vi "ConfigureDlg.vi"(8 "error in (no error)":errorcluster, 11 "RoomAlert in":refnum<class "RoomAlert.lvclass">) -> (0 "error out":errorcluster, 2 "Changed":bool, 3 "RoomAlert out":refnum<class "RoomAlert.lvclass">)   [LabVIEW 2018, in "SensorPlugins.lvlib" / "RoomAlert.lvclass"]
doc: "Configure the instrument using the provided panel and saves the instruments configuration to file, a new file, or cancels the entire operation."
uses:
  RoomAlert.lvclass
  C:/Program Files/National Instruments/LabVIEW 2018/user.lib/NIST/BaseClasses/BasePlugin_class/BasePlugin.lvclass
  TypeDefinitions/RoomAlertControls.ctl
  TypeDefinitions/MeasurementControls.ctl
  <userlib>/NIST/BaseClasses/BasePlugin_class/BasePlugin.lvclass/BasePlugin.ctl
  <userlib>/NIST/BaseClasses/BasePlugin_class/Accessors/Read PluginIniFilePath.vi
  <userlib>/NIST/BaseClasses/BasePlugin_class/Accessors/Write PluginIniFilePath.vi
  <vilib>/Utility/config.llb/NI_LVConfig.lvlib
panel:
  in  "Refresh Measurements Array":bool
  in  "MeasurementCluster":T1={"Measurement RefreshTime (ms)"=1000, "Measurement Name"="Sensor.RoomAlert0", "Timeout(ms)"=1000, "Amber Warning Light Configuration"={"Warning Temperture (Degrees C)"=0.0, "Temperature Delta (Degrees C/Minute)"=0.0, "Time Window (Minutes)"=0.0}} {"Amber Warning Light Configuration"."Time Window (Minutes)" min=0.0; "Timeout(ms)" min=5000; "Measurement RefreshTime (ms)" min=1000}
  in  "RoomAlert Device":T2 {"Measurements To Read Array" items=["Model ID", "Alarm Message", "Internal Temp F", "Internal Temp C", "Digital Sensor 1 Temp F", "Digital Sensor 1 Temp C", "Digital Sensor 2 Temp F", "Digital Sensor 2 Temp C", "Digital Sensor 3 Temp F", "Digital Sensor 3 Temp C", "Digital Switch 1", "Digital Switch 2", "Digital Switch 3", "Digital Switch 4", "Relay"]}
  in  "btnSaveAs":bool
  in  "btnSave":bool
  in  "btnCancel":bool
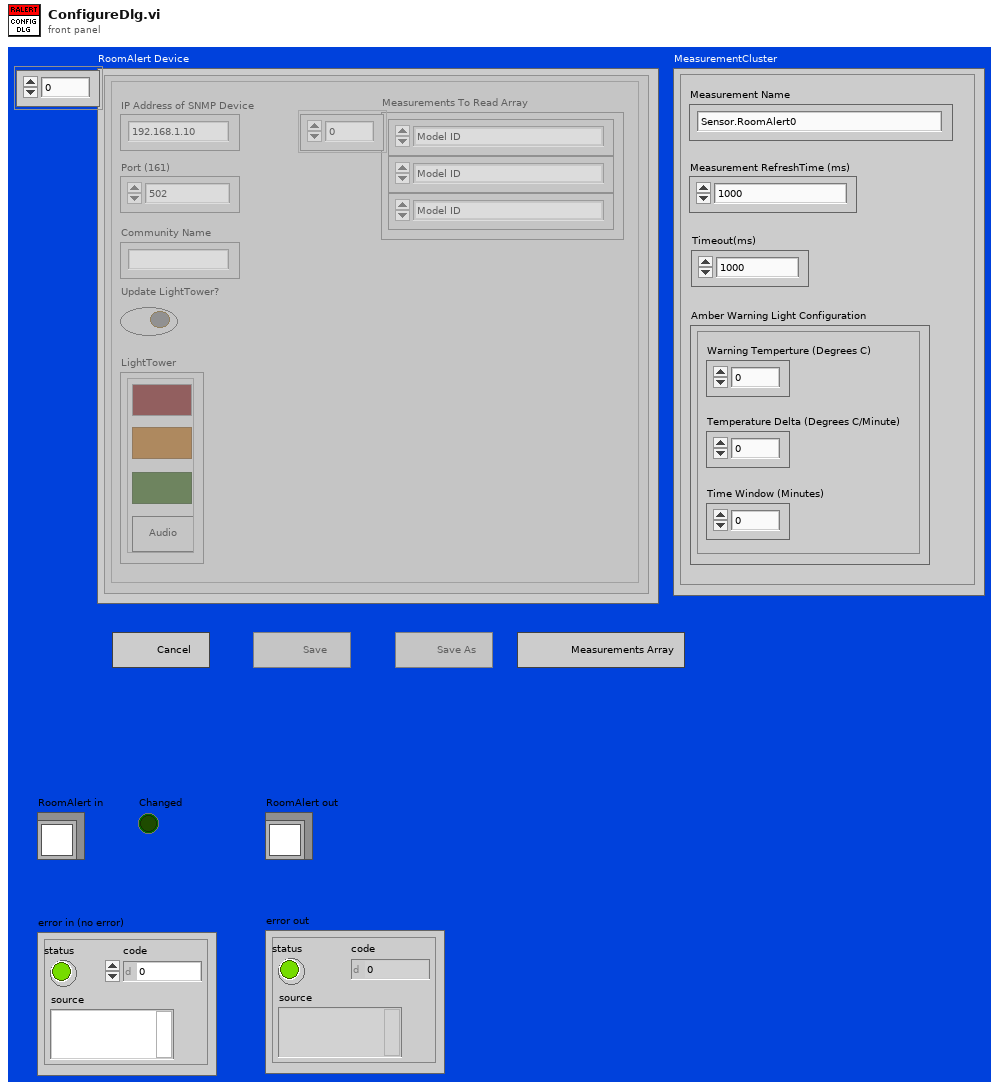
[diagram p1: front panel]
types:
  T1 = typedef "SensorPlugins.lvlib/RoomAlert.lvclass/MeasurementControls.ctl" = cluster{"Measurement RefreshTime (ms)":u32, "Measurement Name":string, "Timeout(ms)":i32, "Amber Warning Light Configuration":cluster{"Warning Temperture (Degrees C)":dbl, "Temperature Delta (Degrees C/Minute)":dbl, "Time Window (Minutes)":dbl}}
  T2 = typedef "SensorPlugins.lvlib/RoomAlert.lvclass/RoomAlertControls.ctl" = cluster{"Connected?":bool, "IP Address of SNMP Device":string, "Port (161)":u16, "Community Name":string, "Measurements To Read Array":u16[], "Update LightTower?":bool, "LightTower":cluster{"Red":bool, "Amber":bool, "Green":bool, "Audio":bool}, "RoomAlert Model ID":string, "Sensor OID Numbers":string[][], "Sensor Light Tower OID Numbers":string[][]}[]
  T3 = enum32{"Invalid", "Default", "Floating", "Floating/Auto-Hide", "Modal"}
  T4 = enum32{"Invalid", "Standard", "Closed", "Hidden", "Minimized", "Maximized"}
  T5 = enum8{"Enabled", "Disabled", "Disabled and Grayed Out"}
  T6 = cluster{"Connected?":bool, "IP Address of SNMP Device":string, "Port (161)":u16, "Community Name":string, "Measurements To Read Array":u16[], "Update LightTower?":bool, "LightTower":cluster{"Red":bool, "Amber":bool, "Green":bool, "Audio":bool}, "RoomAlert Model ID":string, "Sensor OID Numbers":string[][], "Sensor Light Tower OID Numbers":string[][]}
  T7 = typedef "NI_LVConfig.lvlib/Config Data RefNum.ctl" = refnum<k1>
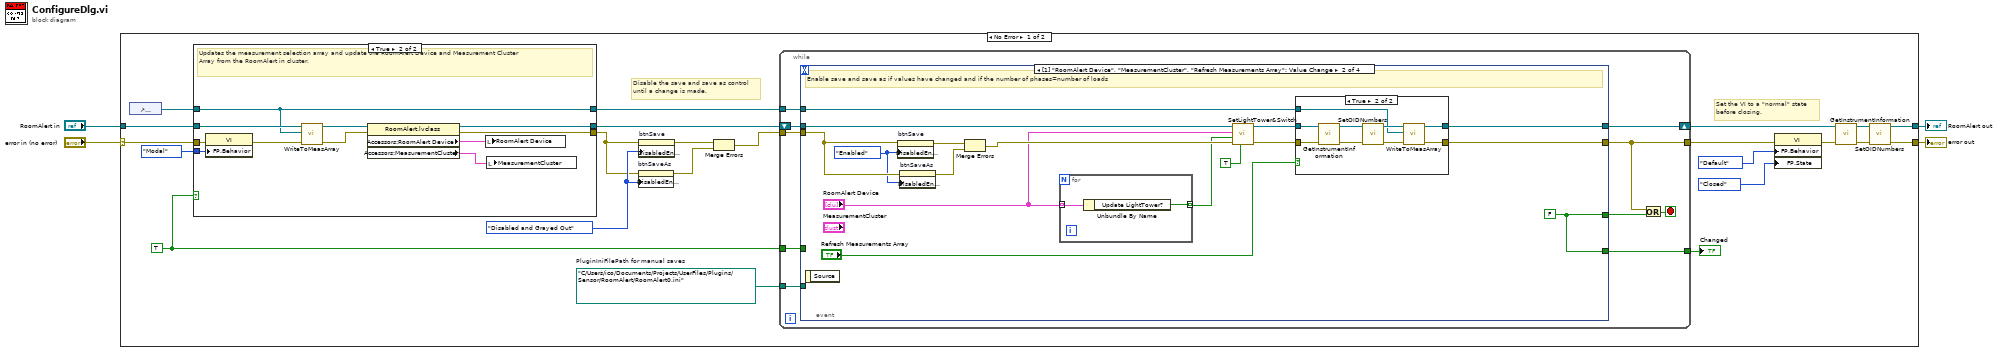
[diagram p0: block diagram]
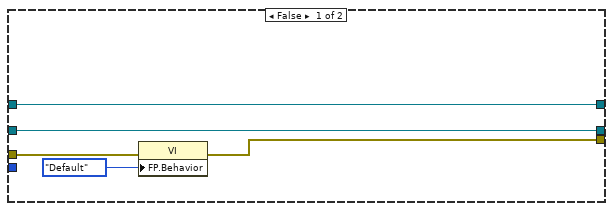
[diagram p2: hidden frame]
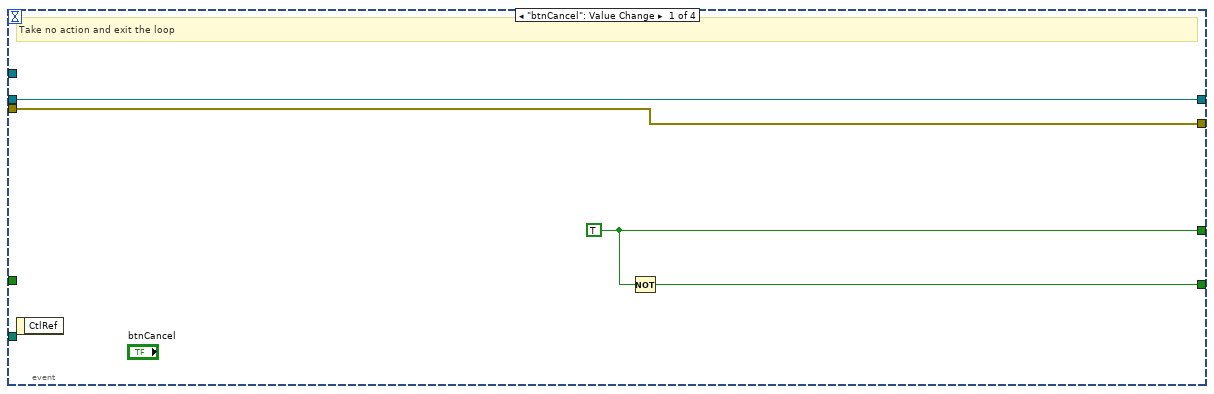
[diagram p3: hidden frame]
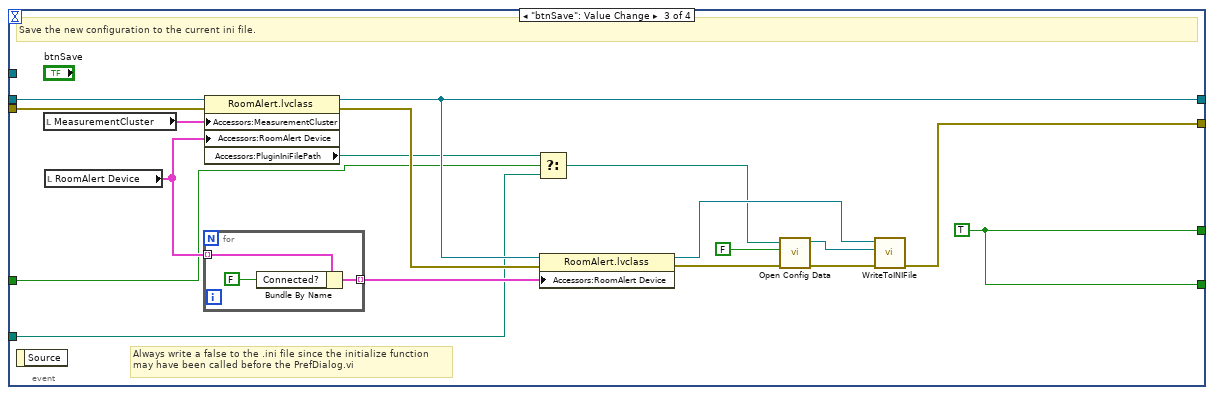
[diagram p5: hidden frame]
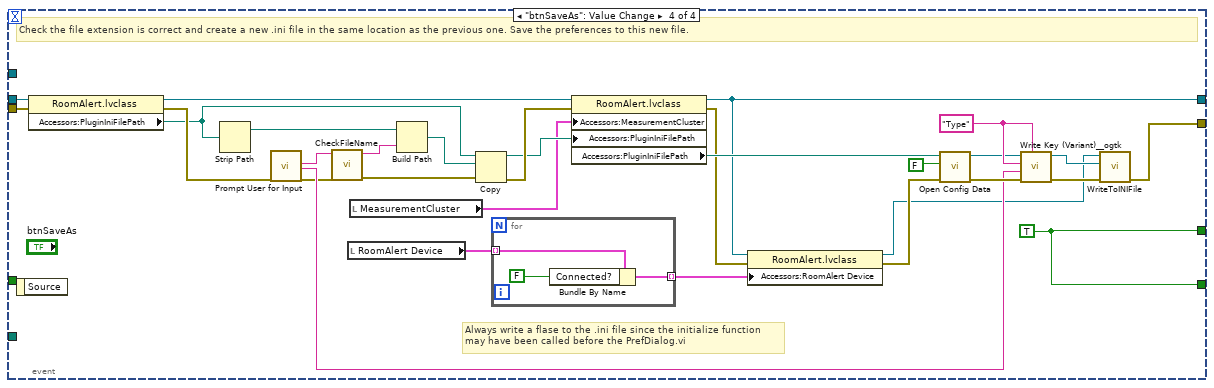
[diagram p6: hidden frame]
diagram:
  n1 = case shown="No Error" "error in (no error)" {
    selector: "error in (no error)" -> [w14 w141]
    tunnel: [w12 w142] -> w2
    tunnel: [w11 w141] -> w1
    tunnel: "RoomAlert in" -> [w15 w142]
    frame No Error {
      w13 = TRUE ("Read from PropertyNode")
      w22 = T5."Disabled and Grayed Out" ("Disabled")
      w19 = path "C:/Users/ico/Documents/Projects/UserFiles/Plugins/Sensor/RoomAlert/RoomAlert0.ini"  # PluginIniFilePath for manual saves
      # "Set the VI to a \"normal\" state\nbefore closing."
      # "Disable the save and save as control\nuntil a change is made."
      n2 = control-ref of="RoomAlert Device"() -> (w5:refnum<vi>)
      n3 = case shown="True" w13 {
        tunnel: T3."Modal" ("Front Panel Window:Behavior") -> [_ w43]
        tunnel: [w32 w42] -> w25
        tunnel: [w30 w41] -> w21
        tunnel: w15 -> [w32 w40]
        tunnel: w14 -> [w31 w39]
        tunnel: [w28 w33] -> w6
        tunnel: w5 -> [w28 w33]
        frame False {
          n4 = property class="VI"(error in=w31, "FP.Behavior"=T3."Default" ("Front Panel Window:Behavior")) -> (error out=w30:errorcluster)  [unwired: 1 in, 1 out]
        }
        frame True {
          # "Updates the measurement selection array and update the RoomAlert Device and Measurement Cluster\nArray from the RoomAlert in cluster."
          n5 = property class="VI"(error in=w39, "FP.Behavior"=w43) -> (error out=w38:errorcluster)  [unwired: 1 in, 1 out]
          n6 = call-dynamic "WriteToMeasArray.vi"("error in (no error)"=w38, "RoomAlert Device Reference"=w33, "RoomAlert in"=w40) -> ("error out"=w36:errorcluster, "RoomAlert out"=w37:refnum<class "RoomAlert.lvclass">)  [unwired: 7 in]
          n7 = property class="RoomAlert.lvclass"(reference=w37, error in=w36) -> (reference out=w42:refnum<class "RoomAlert.lvclass">, error out=w41:errorcluster, "Accessors:RoomAlert Device"=w35:T2, "Accessors:MeasurementCluster"=w34:T1)
          n8 = local write "RoomAlert Device"(w35) -> ()
          n9 = local write "MeasurementCluster"(w34) -> ()
        }
      }
      n10 = property on="btnSaveAs" class="Bool"(error in=w21, "DisabledEnum"=w22) -> (error out=w23:errorcluster)  [unwired: 1 in, 1 out]
      n11 = property on="btnSave" class="Bool"(error in=w21, "DisabledEnum"=w22) -> (error out=w24:errorcluster)  [unwired: 1 in, 1 out]
      n12 = Merge Errors(w24, w23) -> (w20:errorcluster)
      n13 = while {
        shift-right: [w52] -> w7
        shift-left: w25 -> [w53]
        tunnel: w20 -> [w51]
        tunnel: [w48] -> w18
        tunnel: [w50] -> w16
        tunnel: w19 -> [w46]
        tunnel: w13 -> [w45]
        tunnel: w6 -> [w44]
        stop <- w49 stop-if-true
        n14 = event shown="[1] \"RoomAlert Device\", \"MeasurementCluster\", \"Refresh Measurements Array\": Value Change" {
          selector: _ -> [_ _ _ _]
          dyn-events: _ -> [_ _ _ _]
          timeout: _ -> [_ _ _ _]
          tunnel: w53 -> [w57 w67 w102 w123]
          tunnel: [w55 w73 w103 w136] -> w47
          tunnel: [w57 w61 w94 w109] -> w52
          tunnel: w51 -> [w56 w72 w99 w122]
          tunnel: [w56 w60 w100 w134] -> w48
          tunnel: [w54 w73 w103 w136] -> w50
          tunnel: w46 -> [_ _ w91 _]
          tunnel: w45 -> [_ _ w87 _]
          tunnel: w44 -> [_ w59 _ _]
          event "btnCancel": Value Change {
            w55 = TRUE
            # "Take no action and exit the loop"
            n15 = event-data() -> ()  [unwired: 1 in, 1 out]
            n16 = Not(x=w55) -> (.not. x?=w54:bool)
          }
          event "Refresh Measurements Array": Value Change {
            w69 = T5."Enabled" ("Disabled")
            w73 = FALSE
            # "Enable save and save as if values have changed and if the number of phases=number of loads"
            n17 = event-data() -> ()  [unwired: 1 in, 1 out]
            n18 = property on="btnSave" class="Bool"(error in=w72, "DisabledEnum"=w69) -> (error out=w70:errorcluster)  [unwired: 1 in, 1 out]
            n19 = property on="btnSaveAs" class="Bool"(error in=w72, "DisabledEnum"=w69) -> (error out=w71:errorcluster)  [unwired: 1 in, 1 out]
            n20 = Merge Errors(w70, w71) -> (w68:errorcluster)
            n21 = for {
              tunnel: "RoomAlert Device" -> [w86] mode=indexing
              tunnel: [w85] -> w65 mode=indexing
              n22 = Unbundle By Name(w86) -> ("Update LightTower?"=w85:bool)
            }
            n23 = call-dynamic "SetLightTower&Switch.vi"("Supress Match Error (F)"=TRUE, "error in (no error)"=w68, "UpdateValue? (F)"=w65, "RoomAlert Device"="RoomAlert Device", "RoomAlert in"=w67) -> ("error out"=w63:errorcluster, "RoomAlert out"=w62:refnum<class "RoomAlert.lvclass">)  [unwired: 5 in]
            n24 = case shown="True" "Refresh Measurements Array" {
              tunnel: w63 -> [w75 w82]
              tunnel: w62 -> [w74 w81]
              tunnel: [w74 w78] -> w61
              tunnel: [w75 w77] -> w60
              tunnel: w59 -> [_ w76]
              frame False {
              }
              frame True {
                n25 = call "GetInstrumentInformation.vi"("error in (no error)"=w82, "RoomAlert in"=w81) -> ("error out"=w84:errorcluster, "RoomAlert out"=w83:refnum<class "RoomAlert.lvclass">)  [unwired: 7 in, 1 out]
                n26 = call "SetOIDNumbers.vi"("error in (no error)"=w84, "RoomAlert in"=w83) -> ("error out"=w80:errorcluster, "RoomAlert out"=w79:refnum<class "RoomAlert.lvclass">)  [unwired: 8 in]
                n27 = call-dynamic "WriteToMeasArray.vi"("error in (no error)"=w80, "RoomAlert Device Reference"=w76, "RoomAlert in"=w79) -> ("error out"=w77:errorcluster, "RoomAlert out"=w78:refnum<class "RoomAlert.lvclass">)  [unwired: 7 in]
              }
            }
          }
          event "btnSave": Value Change {
            w103 = TRUE
            # "Always write a false to the .ini file since the initialize function\nmay have been called before the PrefDialog.vi"
            # "Save the new configuration to the current ini file."
            n28 = event-data() -> ()  [unwired: 1 in, 1 out]
            n29 = local read "MeasurementCluster"() -> (w88:T1)
            n30 = local read "RoomAlert Device"() -> (w89:T2)
            n31 = for {
              tunnel: w89 -> [w106] mode=indexing
              tunnel: [w107] -> w97 mode=indexing
              n32 = Bundle By Name(cluster=w106, "Connected?"=FALSE) -> (w107:T6)
            }
            n33 = property class="RoomAlert.lvclass"(reference=w102, error in=w99, "Accessors:MeasurementCluster"=w88, "Accessors:RoomAlert Device"=w89) -> (reference out=w94:refnum<class "RoomAlert.lvclass">, error out=w98:errorcluster, "Accessors:PluginIniFilePath"=w92:path)
            n34 = Select(t=w92, s=w87, f=w91) -> (s? t:f=w90:path)
            n35 = property class="RoomAlert.lvclass"(reference=w94, error in=w98, "Accessors:RoomAlert Device"=w97) -> (reference out=w93:refnum<class "RoomAlert.lvclass">, error out=w95:errorcluster)
            n36 = call <vilib>:"Open Config Data.vi"("error in (no error)"=w95, "create file if necessary (T)"=FALSE, "configuration file path"=w90) -> ("error out"=w96:errorcluster, "refnum"=w101:T7)  [unwired: 6 in, 1 out]
            n37 = call-dynamic "WriteToINIFile.vi"("error in (no error)"=w96, "Refnum in"=w101, "RoomAlert in"=w93) -> ("error out"=w100:errorcluster)  [unwired: 7 in, 1 out]
          }
          event "btnSaveAs": Value Change {
            w133 = "Type" ("section (optional)")
            w136 = TRUE
            # "Always write a flase to the .ini file since the initialize function\nmay have been called before the PrefDialog.vi"
            # "Check the file extension is correct and create a new .ini file in the same location as the previous one. Save the preferences to this new file."
            n38 = event-data() -> ()  [unwired: 1 in, 1 out]
            n39 = property class="RoomAlert.lvclass"(reference=w123, error in=w122) -> (reference out=w121:refnum<class "RoomAlert.lvclass">, error out=w120:errorcluster, "Accessors:PluginIniFilePath"=w119:path)
            n40 = Strip Path(path=w119) -> (stripped path=w128:path)  [unwired: 1 out]
            n41 = call "Prompt User for Input"("error in (no error)"=w120) -> ("File Name"=w115:string, "PluginType"=w118:string, "error out"=w114:errorcluster)  [unwired: 15 in, 1 out]
            n42 = call "CheckFileName.vi"("Error In"=w114, "File Name in"=w115) -> ("Error Out"=w116:errorcluster, "File Name out"=w117:string)  [unwired: 8 in]
            n43 = local read "RoomAlert Device"() -> (w135:T2)
            n44 = local read "MeasurementCluster"() -> (w113:T1)
            n45 = Build Path(base path=w128, name or relative path=w117) -> (appended path=w127:path)
            n46 = Copy(8:w116, 10:w127, 11:w119) -> (0:w126:errorcluster, 3:w124:path)  [unwired: 2 in, 1 out]
            n47 = for {
              tunnel: w135 -> [w139] mode=indexing
              tunnel: [w140] -> w112 mode=indexing
              n48 = Bundle By Name(cluster=w139, "Connected?"=FALSE) -> (w140:T6)
            }
            n49 = property class="RoomAlert.lvclass"(reference=w121, error in=w126, "Accessors:MeasurementCluster"=w113, "Accessors:PluginIniFilePath"=w124) -> (reference out=w109:refnum<class "RoomAlert.lvclass">, error out=w111:errorcluster, "Accessors:PluginIniFilePath"=w125:path)
            n50 = property class="RoomAlert.lvclass"(reference=w109, error in=w111, "Accessors:RoomAlert Device"=w112) -> (reference out=w108:refnum<class "RoomAlert.lvclass">, error out=w110:errorcluster)
            n51 = call <vilib>:"Open Config Data.vi"("error in (no error)"=w110, "create file if necessary (T)"=FALSE, "configuration file path"=w125) -> ("error out"=w131:errorcluster, "refnum"=w132:T7)  [unwired: 6 in, 1 out]
            n52 = call <userlib>:"Write Key (Variant)__ogtk.vi"("section"=w133, "error in (no error)"=w131, "key-value"=w118, "key (optional)"=w133, "refnum"=w132) -> ("error out"=w130:errorcluster, "refnum out"=w129:T7)  [unwired: 5 in]
            n53 = call-dynamic "WriteToINIFile.vi"("error in (no error)"=w130, "Refnum in"=w129, "RoomAlert in"=w108) -> ("error out"=w134:errorcluster)  [unwired: 7 in, 1 out]
          }
        }
        n54 = Or(x=w48, y=w47) -> (x .or. y?=w49:bool)
      }
      "Changed" <- w16
      n55 = property class="VI"(error in=w18, "FP.Behavior"=T3."Default" ("Front Panel Window:Behavior"), "FP.State"=T4."Closed" ("Front Panel Window:State")) -> (error out=w8:errorcluster)  [unwired: 1 in, 1 out]
      n56 = call "GetInstrumentInformation.vi"("error in (no error)"=w8, "RoomAlert in"=w7) -> ("error out"=w10:errorcluster, "RoomAlert out"=w9:refnum<class "RoomAlert.lvclass">)  [unwired: 7 in, 1 out]
      n57 = call "SetOIDNumbers.vi"("error in (no error)"=w10, "RoomAlert in"=w9) -> ("error out"=w11:errorcluster, "RoomAlert out"=w12:refnum<class "RoomAlert.lvclass">)  [unwired: 8 in]
    }
    frame Error {
    }
  }
  "error out" <- w1
  "RoomAlert out" <- w2
